vi "gSIM.vi"() -> ()   [LabVIEW 2011]
panel:
  out "gSIM":bool
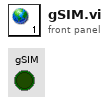
[diagram p1: front panel]
diagram:
